vi "FormatMessageWithValue.vi"(8 "error in":errorcluster, 10 "value":string, 11 "cmd":string) -> (0 "error out":errorcluster, 3 "JSON string":string)   [LabVIEW 2014, in "Raspberry Pi Compatible Compiler for LabVIEW.lvlib" / "RasPiDownloader.lvlib"]
uses:
  RasPiDownloader.lvlib
  MessageWithValueTD.ctl
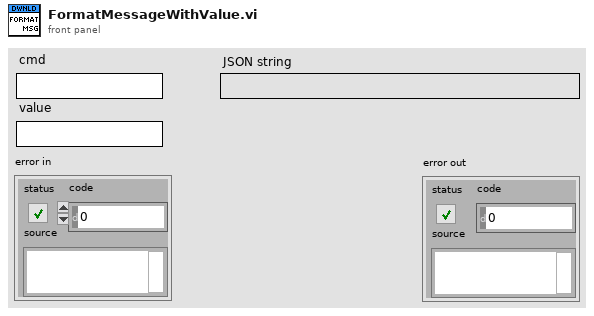
[diagram p1: front panel]
types:
  T1 = typedef "Raspberry Pi Compatible Compiler for LabVIEW.lvlib/RasPiDownloader.lvlib/MessageWithValueTD.ctl" = cluster{"cmd":string, "value":string}
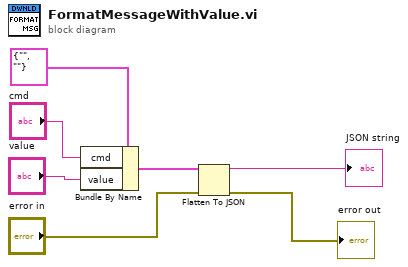
[diagram p0: block diagram]
diagram:
  n1 = Bundle By Name(cluster=T1 {"cmd"="", "value"=""} ("message"), "cmd"="cmd", "value"="value") -> (w4:T1)
  n2 = Flatten To JSON(anything=w4, error in (no error)="error in") -> (JSON string=→"JSON string":string, 11:→"error out":errorcluster)  [unwired: 1 in]
